vi "Convert to API Format.vi"(11 "digital audio protocol settings":T9={"number of channels"=0, "data justification"=enum."Left Justified", "endianness"=enum."LSB First", "channel length"=0, "bit depth"=0, "frame clock rate"=0.0, "bit clock edge sync"=enum."Falling", "master clock rate"=0.0, "Logic Level"=enum."1.2 V", "frame sync edge for channel 0"=enum."Rising", "Channel 0 Offset"=0}) -> (3 "digital protocol settings":T1={"logic level"=enum."3.3 V", "PCM Data Configuration"={"Frame Sync Edge for Channel 0"=enum."Falling", "Channel Count Per Frame"=2, "Channel Length"=32, "Bit Depth"=24, "Channel 0 Offset"=1, "Endianness"=enum."MSB First", "Data Justification"=enum."Left Justified"}, "bit clock rate"=3025000.0, "master clock rate"=3025000.0, "clock mode"=enum."divided clock", "Frame Sync Clock Control"={"Frame Length"=64, "Frame Sync Pulse Width"=32, "Bit Clock Edge  Sync"=enum."Falling"}} {"master clock rate" format="%.4p"; "bit clock rate" format="%.4p"})   [LabVIEW 2023, in "digital audio protocol controls.lvlib"]
uses:
  digital audio protocol controls.lvlib
  controls/digital serial gen settings.ctl
  <vilib>/PDM Acquisition Toolkit/shared/controls/PCM Data Justification.ctl
  <vilib>/PDM Acquisition Toolkit/shared/controls/PCM Bit Endianness.ctl
  <vilib>/PDM Acquisition Toolkit/shared/controls/Digital Edge.ctl
  <vilib>/PDM Acquisition Toolkit/host/Classes/Session/Controls/Logic Levels.ctl
  service/generation/controls/digital protocol settings.ctl
  <vilib>/PDM Acquisition Toolkit/shared/controls/PCM Data Format Configuration.ctl
  <vilib>/PDM Acquisition Toolkit/shared/controls/clock mode.ctl
  <vilib>/PDM Acquisition Toolkit/shared/controls/PCM Frame Sync Control.ctl
  <vilib>/PDM Acquisition Toolkit/shared/PDM Shared.lvlib
  <vilib>/PDM Acquisition Toolkit/host/Classes/Session/DecoderSession.lvclass
  service/generation/controls/AudioGenTypeDefs.lvlib
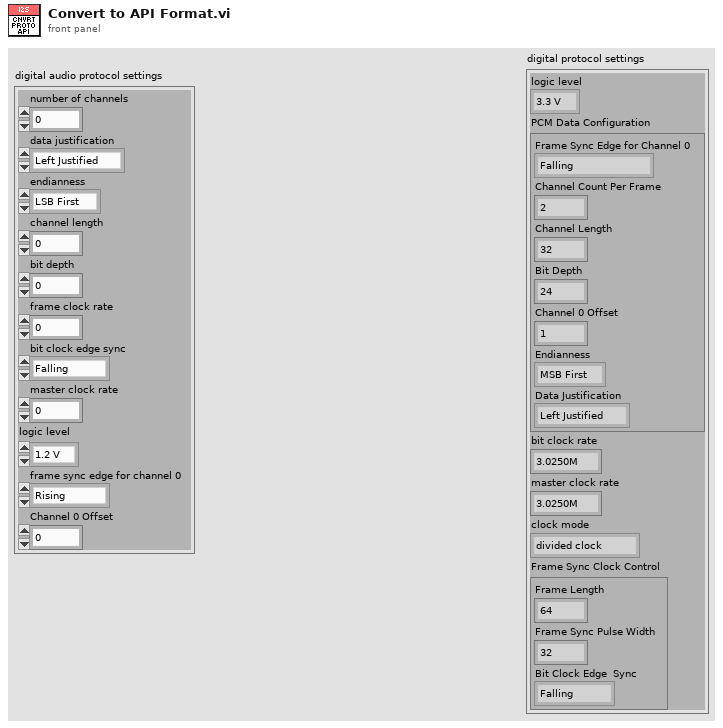
[diagram p1: front panel]
types:
  T1 = typedef "AudioGenTypeDefs.lvlib/digital protocol settings.ctl" = cluster{"logic level":T2, "PCM Data Configuration":T3, "bit clock rate":sgl, "master clock rate":sgl, "clock mode":T7, "Frame Sync Clock Control":T8}
  T2 = typedef "PDM Acquisition Class Library.lvlib/DecoderSession.lvclass/Logic Levels.ctl" = enum16{"3.3 V", "1.8 V", "1.2 V"}
  T3 = typedef "PDM Shared.lvlib/PCM Data Format Configuration.ctl" = cluster{"Frame Sync Edge for Channel 0":T4, "Channel Count Per Frame":u8, "Channel Length":u16, "Bit Depth":u8, "Channel 0 Offset":u16, "Endianness":T5, "Data Justification":T6}
  T4 = typedef "PDM Shared.lvlib/Digital Edge.ctl" = enum8{"Rising", "Falling"}
  T5 = typedef "PDM Shared.lvlib/PCM Bit Endianness.ctl" = enum16{"MSB First", "LSB First"}
  T6 = typedef "PDM Shared.lvlib/PCM Data Justification.ctl" = enum16{"Left Justified", "Right Justified"}
  T7 = typedef "PDM Shared.lvlib/clock mode.ctl" = enum16{"divided clock", "DDS"}
  T8 = typedef "PDM Shared.lvlib/PCM Frame Sync Control.ctl" = cluster{"Frame Length":u16, "Frame Sync Pulse Width":u16, "Bit Clock Edge  Sync":T4}
  T9 = typedef "digital serial gen settings.ctl" = cluster{"number of channels":u32, "data justification":T6, "endianness":T5, "channel length":u32, "bit depth":u32, "frame clock rate":dbl, "bit clock edge sync":T4, "master clock rate":dbl, "Logic Level":T2, "frame sync edge for channel 0":T4, "Channel 0 Offset":u32}
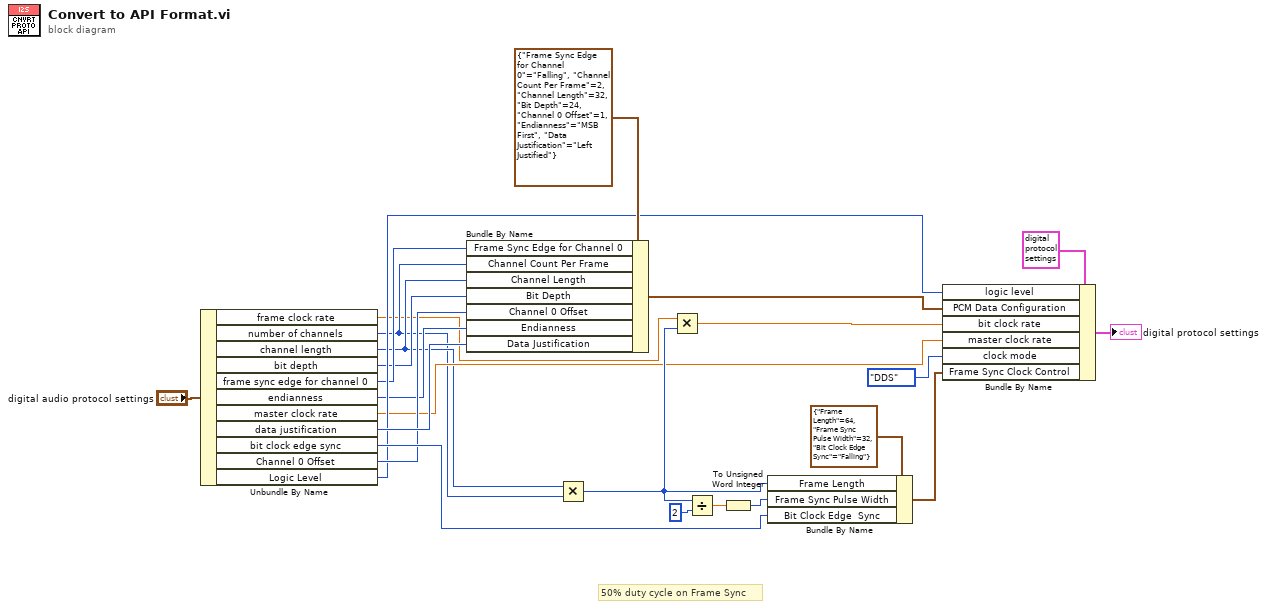
[diagram p0: block diagram]
diagram:
  # "50% duty cycle on Frame Sync"
  n1 = Unbundle By Name("digital audio protocol settings") -> ("frame clock rate"=w4:dbl, "number of channels"=w5:u32, "channel length"=w6:u32, "bit depth"=w7:u32, "frame sync edge for channel 0"=w8:T4, "endianness"=w9:T5, "master clock rate"=w10:dbl, "data justification"=w14:T6, "bit clock edge sync"=w13:T4, "Channel 0 Offset"=w12:u32, "Logic Level"=w11:T2)
  n2 = Bundle By Name(cluster=T3 {"Frame Sync Edge for Channel 0"=enum."Falling", "Channel Count Per Frame"=2, "Channel Length"=32, "Bit Depth"=24, "Channel 0 Offset"=1, "Endianness"=enum."MSB First", "Data Justification"=enum."Left Justified"} ("PCM Data Configuration"), "Frame Sync Edge for Channel 0"=w8, "Channel Count Per Frame"=w5, "Channel Length"=w6, "Bit Depth"=w7, "Channel 0 Offset"=w12, "Endianness"=w9, "Data Justification"=w14) -> (w18:T3)
  n3 = Multiply(x=w6, y=w5) -> (x*y=w20:u32)
  n4 = Multiply(x=w4, y=w20) -> (x*y=w17:dbl)
  n5 = Divide(x=w20, y=u16 2) -> (x/y=w22:dbl)
  n6 = To Unsigned Word Integer(number=w22) -> (unsigned 16bit integer=w21:u16)
  n7 = Bundle By Name(cluster=T8 {"Frame Length"=64, "Frame Sync Pulse Width"=32, "Bit Clock Edge  Sync"=enum."Falling"} ("Frame Sync Clock Control"), "Frame Length"=w20, "Frame Sync Pulse Width"=w21, "Bit Clock Edge  Sync"=w13) -> (w16:T8)
  n8 = Bundle By Name(cluster=T1 {"logic level"=enum."3.3 V", "PCM Data Configuration"={"Frame Sync Edge for Channel 0"=enum."Falling", "Channel Count Per Frame"=2, "Channel Length"=32, "Bit Depth"=24, "Channel 0 Offset"=1, "Endianness"=enum."MSB First", "Data Justification"=enum."Left Justified"}, "bit clock rate"=3025000.0, "master clock rate"=3025000.0, "clock mode"=enum."divided clock", "Frame Sync Clock Control"={"Frame Length"=64, "Frame Sync Pulse Width"=32, "Bit Clock Edge  Sync"=enum."Falling"}} ("digital protocol settings"), "logic level"=w11, "PCM Data Configuration"=w18, "bit clock rate"=w17, "master clock rate"=w10, "clock mode"=clock_mode."DDS", "Frame Sync Clock Control"=w16) -> (→"digital protocol settings":T1)
